vi "ReplaceValue.vi"(8 "新值":string="dfd", 9 "键":string="d", 10 "添加？":bool, 11 "键值串":string="[a=a][b=b][c=c]") -> (3 "替换后的键值串":string)   [LabVIEW 2020, in "Curve Editor.lvlib" / "Key Value.lvlib"]
uses:
  Key Value.lvlib
panel:
  # "替换键值串中某个键的值，如果这个键不存在可以选择是否添加"
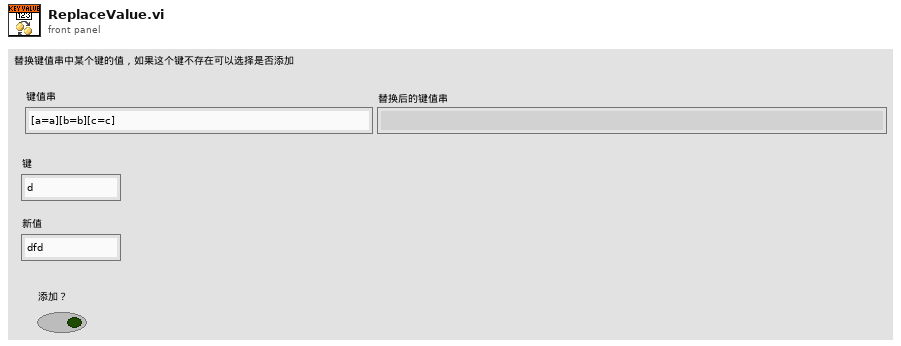
[diagram p1: front panel]
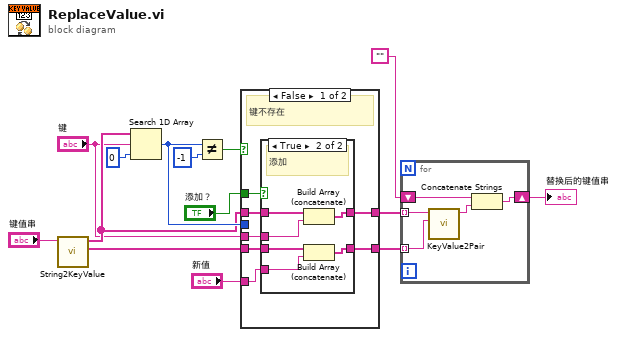
[diagram p0: block diagram]
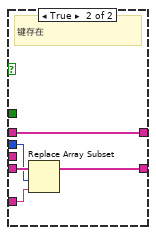
[diagram p3: hidden frame]
diagram:
  n1 = call "String2KeyValue.vi"("健值对字符串"="键值串") -> ("值数组"=w10:string[], "键数组"=w4:string[])  [unwired: 9 in]
  n2 = Search 1D Array(1D array=w4, element="键", start index (0)=0 ("开始索引(0)")) -> (index of element=w9:i32)
  n3 = Not Equal?(x=w9, y=-1) -> (x != y?=w11:bool)
  n4 = case shown="False" w11 {
    tunnel: w10 -> [w18 w34]
    tunnel: w9 -> [_ w33]
    tunnel: "新值" -> [w15 w32]
    tunnel: [w17 w31] -> w7
    tunnel: w4 -> [w20 w30]
    tunnel: [w19 w30] -> w3
    tunnel: "添加？" -> [w21 _]
    tunnel: "键" -> [w16 _]
    frame False {
      # "键不存在"
      n5 = case shown="True" w21 {
        tunnel: w20 -> [w23 w29]
        tunnel: [w23 w27] -> w19
        tunnel: w18 -> [w22 w26]
        tunnel: [w22 w24] -> w17
        tunnel: w16 -> [_ w28]
        tunnel: w15 -> [_ w25]
        frame False {
          # "不添加"
        }
        frame True {
          # "添加"
          n6 = Build Array (concatenate)(w29, w28) -> (w27:string[])
          n7 = Build Array (concatenate)(w26, w25) -> (w24:string[])
        }
      }
    }
    frame True {
      # "键存在"
      n8 = Replace Array Subset(array=w34, new element=w32, index=w33) -> (w31:string[])
    }
  }
  n9 = for {
    tunnel: w3 -> [w39] mode=indexing
    tunnel: w7 -> [w38] mode=indexing
    shift-right: [w35] -> w5
    shift-left: "" -> [w37]
    n10 = call "KeyValue2Pair.vi"("值"=w38, "键"=w39) -> ("键值对"=w36:string)  [unwired: 9 in]
    n11 = Concatenate Strings(w37, w36) -> (w35:string)
  }
  "替换后的键值串" <- w5
